vi "Keithley2400series_Start2.vi"(4 "Serial Configuration":T1={"Baud Rate"=9600, "Parity"=0, "Data Bits"=8, "Stop Bits"=10, "Flow Control"=0} {"Flow Control" items=["None", "XON/XOFF", "RTS/CTS", "XON/XOFF & RTS/CTS", "DTR/DSR", "XON/XOFF & DTR/DSR"]; "Stop Bits" items=["1.0"=10, "1.5"=15, "2.0"=20]; "Data Bits" items=["7"=7, "8"=8]; "Parity" items=["None", "Odd", "Even", "Mark", "Space"]; "Baud Rate" items=["300"=300, "600"=600, "1200"=1200, "2400"=2400, "4800"=4800, "9600"=9600, "19200"=19200]}, 6 "Source Mode  (0: Voltage) in":u16(ring) items=["Voltage", "Current"], 7 "4W on":bool, 9 "Ограничение":dbl format="%.2f", 10 "Выход":dbl, 11 "VISA Refnum in":refnum<visa-resource-name>) -> (0 "error out":errorcluster, 2 "MEAS:Out":string, 3 "VISA Refnum out":refnum<visa-resource-name>, 5 "MEAS mode 0,Volt":dbl)   [LabVIEW 2014]
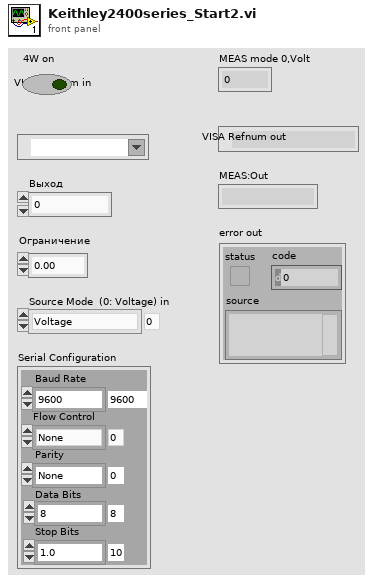
[diagram p1: front panel]
types:
  T1 = cluster{"Baud Rate":u32, "Parity":u16, "Data Bits":u16, "Stop Bits":u16, "Flow Control":u16}
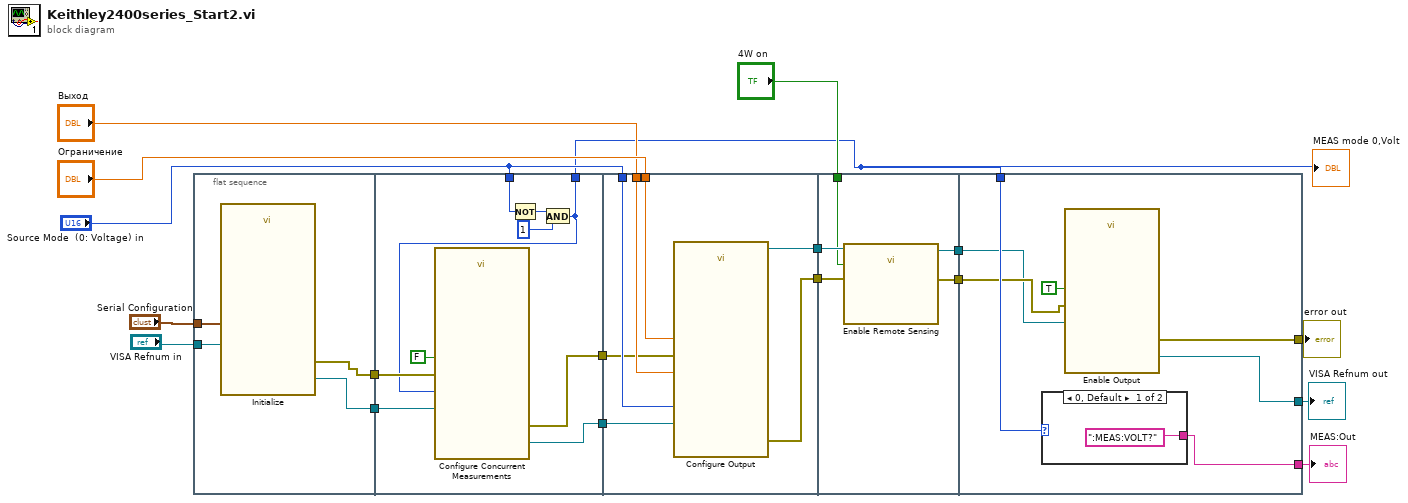
[diagram p0: block diagram]
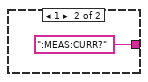
[diagram p2: hidden frame]
diagram:
  n1 = flat-sequence {
    tunnel: "VISA Refnum in" -> [w22]
    tunnel: "Serial Configuration" -> [w21]
    tunnel: [w20] -> w18
    tunnel: [w19] -> w17
    tunnel: "Source Mode  (0: Voltage) in" -> [w28]
    tunnel: [w27] -> w16
    tunnel: [w26] -> w15
    tunnel: w18 -> [w25]
    tunnel: w17 -> [w24]
    tunnel: [w23] -> w1
    tunnel: "Ограничение" -> [w38]
    tunnel: "Выход" -> [w37]
    tunnel: "Source Mode  (0: Voltage) in" -> [w36]
    tunnel: w16 -> [w35]
    tunnel: w15 -> [w34]
    tunnel: [w33] -> w14
    tunnel: [w32] -> w13
    tunnel: w14 -> [w43]
    tunnel: w13 -> [w42]
    tunnel: [w41] -> w12
    tunnel: [w40] -> w11
    tunnel: "4W on" -> [w39]
    tunnel: w1 -> [w49]
    tunnel: [w48] -> w5
    tunnel: [w47] -> w4
    tunnel: [w46] -> w3
    tunnel: w12 -> [w45]
    tunnel: w11 -> [w44]
    frame #0 {
      n2 = call "Initialize.vi"("Serial Configuration"=w21, "VISA resource name"=w22) -> ("error out"=w19:errorcluster, "VISA resource name out"=w20:refnum<visa-resource-name>)  [unwired: 8 in]
    }
    frame #1 {
      n3 = Not(x=w28) -> (.not. x?=w30:u16)
      n4 = And(x=w30, y=u16 1) -> (x .and. y?=w23:u16)
      n5 = call "Configure Concurrent Measurements.vi"("error in (no error)"=w24, "Measurement Selection (3: Volts, Current)"=w23, "Enable Concurrent Measurements (F: Disable)"=FALSE, "VISA resource name"=w25) -> ("error out"=w26:errorcluster, "VISA resource name out"=w27:refnum<visa-resource-name>)  [unwired: 6 in]
    }
    frame #2 {
      n6 = call "Configure Output.vi"("Source Mode  (0: Voltage)"=w36, "error in (no error)"=w34, "Compliance  Level (0.1)"=w38, "Output Level (0)"=w37, "VISA resource name"=w35) -> ("error out"=w32:errorcluster, "VISA resource name out"=w33:refnum<visa-resource-name>)  [unwired: 5 in]
    }
    frame #3 {
      n7 = call "Enable Remote Sensing.vi"("error in (no error)"=w42, "Enable Remote Sensing (T: Enable)"=w39, "VISA resource name"=w43) -> ("error out"=w41:errorcluster, "VISA resource name out"=w40:refnum<visa-resource-name>)  [unwired: 7 in]
    }
    frame #4 {
      n8 = case shown="0, Default" w49 {
        tunnel: [":MEAS:VOLT?" ":MEAS:CURR?"] -> w46
        frame 0, Default {
        }
        frame 1 {
        }
      }
      n9 = call "Enable Output.vi"("error in (no error)"=w45, "Enable Output (T: Enable)"=TRUE, "VISA resource name"=w44) -> ("error out"=w48:errorcluster, "VISA resource name out"=w47:refnum<visa-resource-name>)  [unwired: 7 in]
    }
  }
  "error out" <- w5
  "VISA Refnum out" <- w4
  "MEAS:Out" <- w3
  "MEAS mode 0,Volt" <- w1
